vi "Flattening of SGL arrays.vi"() -> ()   [LabVIEW 2017]
uses:
  JSONtext.lvlib
panel:
  in  "enable LabVIEW extensions?":bool=TRUE
  in  "Boolean":bool
  out "time":dbl format="%#_3p"
  out "JSON string":string
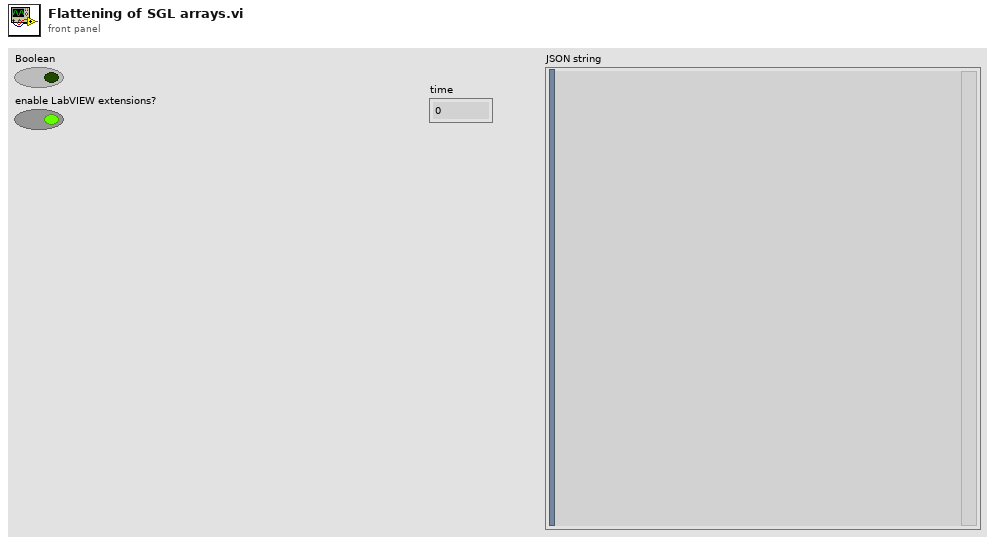
[diagram p1: front panel]
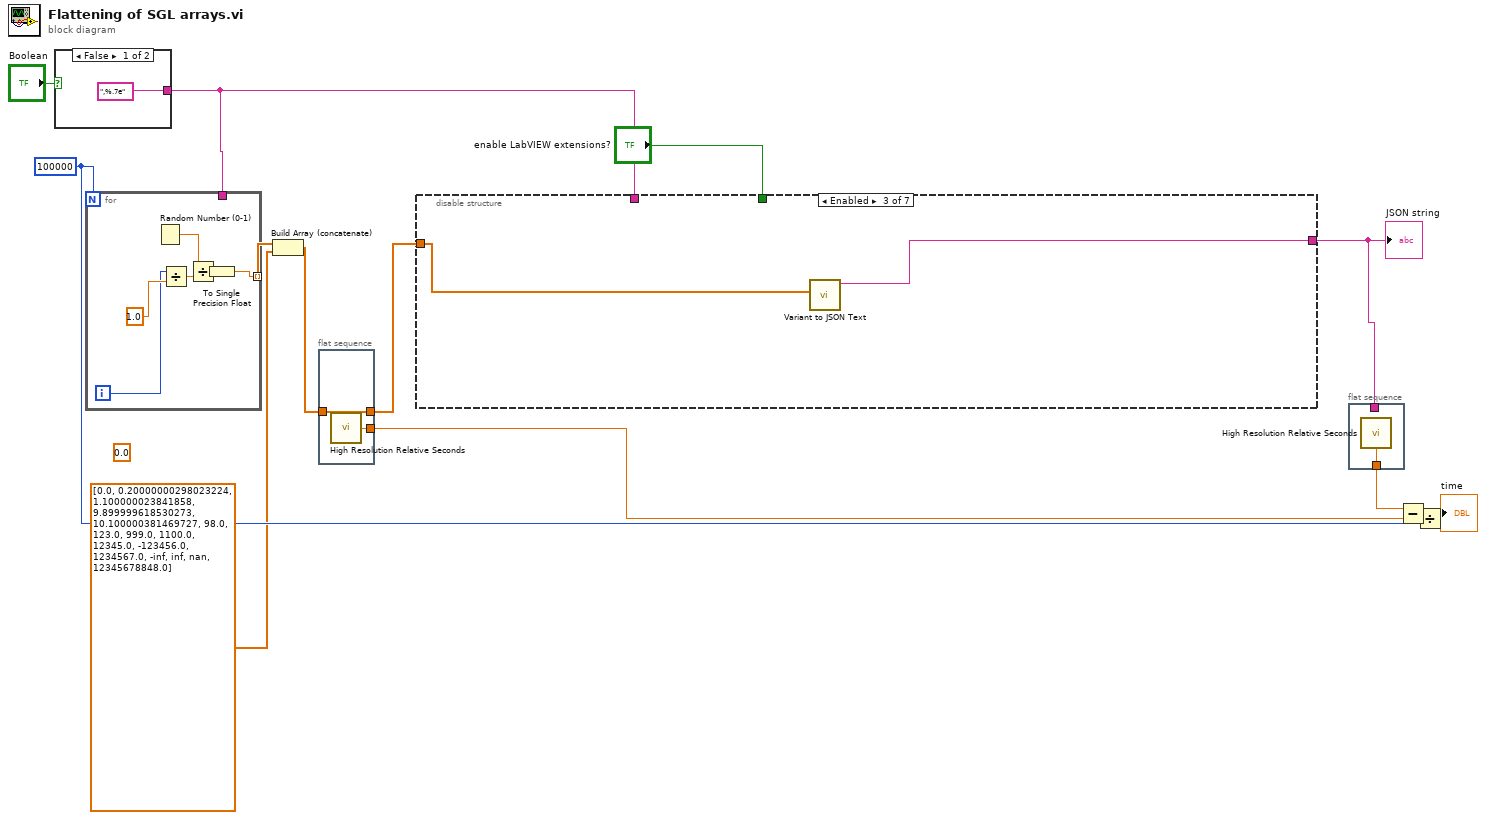
[diagram p0: block diagram]
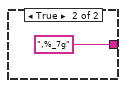
[diagram p2: hidden frame]
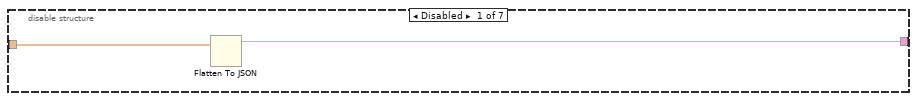
[diagram p3: hidden frame]
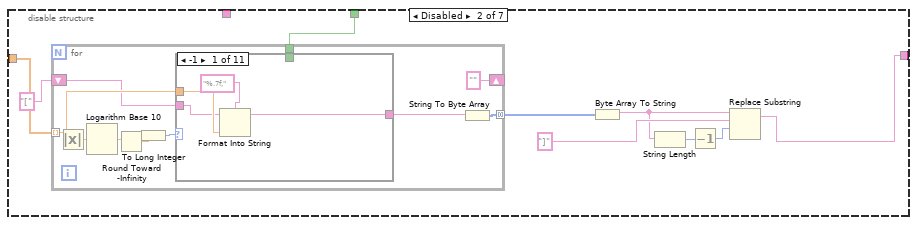
[diagram p4: hidden frame]
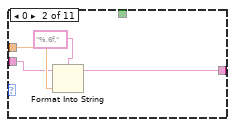
[diagram p5: hidden frame]
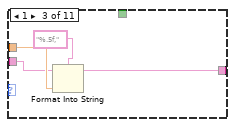
[diagram p6: hidden frame]
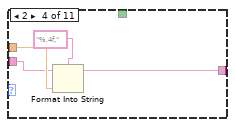
[diagram p7: hidden frame]
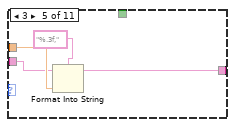
[diagram p8: hidden frame]
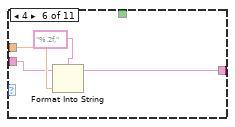
[diagram p9: hidden frame]
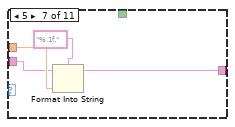
[diagram p10: hidden frame]
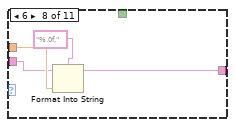
[diagram p11: hidden frame]
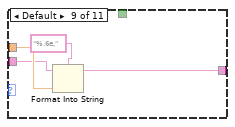
[diagram p12: hidden frame]
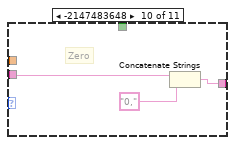
[diagram p13: hidden frame]
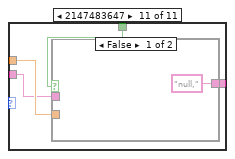
[diagram p14: hidden frame]
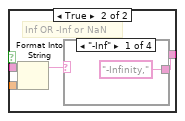
[diagram p15: hidden frame]
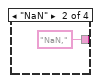
[diagram p16: hidden frame]
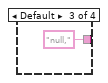
[diagram p17: hidden frame]
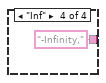
[diagram p18: hidden frame]
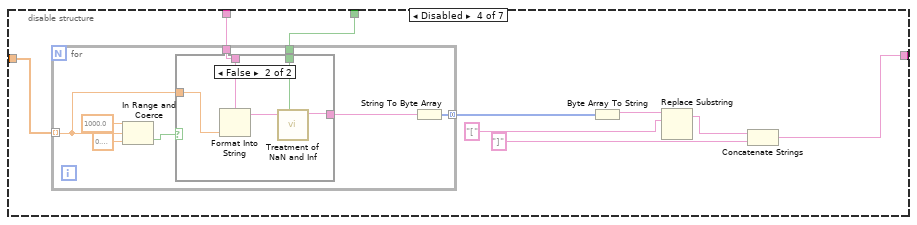
[diagram p19: hidden frame]
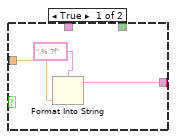
[diagram p20: hidden frame]
diagram:
  (unwired) sgl 0.0
  w6 = 100000
  n1 = case shown="False" "Boolean" {
    tunnel: [",%.7e" ("format string") ",%_7g" ("format string")] -> w3
    frame False {
    }
    frame True {
    }
  }
  n2 = for {
    N: w6 -> [_]
    tunnel: [w16] -> w10 mode=indexing
    tunnel: w3 -> [_]
    i -> [w17]
    n3 = Random Number (0-1)() -> (number: 0 to 1=w19:dbl)
    n4 = Divide(x=w17, y=1.0) -> (x/y=w20:dbl)
    n5 = Divide(x=w19, y=w20) -> (x/y=w18:dbl)
    n6 = To Single Precision Float(number=w18) -> (single precision float=w16:sgl)
  }
  n7 = Build Array (concatenate)(w10, sgl[] [0.0, 0.2, 1.1, 9.9, 10.1, 98.0, 123.0, 999.0, 1100.0, 12345.0, -123456.0, 1234567.0, -inf, inf, nan, 12345679000.0]) -> (w5:sgl[])
  n8 = flat-sequence {
    tunnel: [w23] -> w11
    tunnel: w5 -> [w22]
    tunnel: [w22] -> w9
    frame #0 {
      n9 = call <vilib>:"High Resolution Relative Seconds.vi"() -> ("relative seconds"=w23:dbl)
    }
  }
  n10 = disable-structure shown="Enabled" {
    disable-tunnel: [w25 w30 w97 w101 w126 w141 w164] -> w13
    disable-tunnel: w9 -> [w24 w34 w98 w107 w132 w151 w169]
    disable-tunnel: w3 -> [_ _ _ w100 w125 w139 _]
    disable-tunnel: "enable LabVIEW extensions?" -> [_ w32 _ w99 w124 _ _]
    frame Disabled {
      n11 = Flatten To JSON(anything=w24) -> (JSON string=w25:string)  [unwired: 2 in, 1 out]
    }
    frame Disabled {
      n12 = for {
        tunnel: w34 -> [w42] mode=indexing
        tunnel: [w44] -> w33 mode=concatenating
        tunnel: w32 -> [w43]
        shift-right: [""] -> _
        shift-left: "[" -> [w37]
        n13 = Absolute Value(x=w42) -> (abs(x)=w38:sgl)
        n14 = Logarithm Base 10(1:w38) -> (0:w41:sgl)
        n15 = Round Toward -Infinity(1:w41) -> (0:w40:sgl)
        n16 = To Long Integer(number=w40) -> (32bit integer=w39:i32)
        n17 = case shown="-1" w39 {
          tunnel: [w48 w52 w56 w60 w64 w68 w72 w76 w79 w82 w87] -> w35
          tunnel: w42 -> [w47 w51 w55 w59 w63 w67 w71 w75 w80 _ w86]
          tunnel: w43 -> [_ _ _ _ _ _ _ _ _ _ w85]
          tunnel: w37 -> [w45 w49 w53 w57 w61 w65 w69 w73 w77 w81 w84]
          frame -1 {
            n18 = Format Into String(format string="%.7f,", initial string=w45, w47) -> (resulting string=w48:string)  [unwired: 1 in, 1 out]
          }
          frame 0 {
            n19 = Format Into String(format string="%.6f,", initial string=w49, w51) -> (resulting string=w52:string)  [unwired: 1 in, 1 out]
          }
          frame 1 {
            n20 = Format Into String(format string="%.5f,", initial string=w53, w55) -> (resulting string=w56:string)  [unwired: 1 in, 1 out]
          }
          frame 2 {
            n21 = Format Into String(format string="%.4f,", initial string=w57, w59) -> (resulting string=w60:string)  [unwired: 1 in, 1 out]
          }
          frame 3 {
            n22 = Format Into String(format string="%.3f,", initial string=w61, w63) -> (resulting string=w64:string)  [unwired: 1 in, 1 out]
          }
          frame 4 {
            n23 = Format Into String(format string="%.2f,", initial string=w65, w67) -> (resulting string=w68:string)  [unwired: 1 in, 1 out]
          }
          frame 5 {
            n24 = Format Into String(format string="%.1f,", initial string=w69, w71) -> (resulting string=w72:string)  [unwired: 1 in, 1 out]
          }
          frame 6 {
            n25 = Format Into String(format string="%.0f,", initial string=w73, w75) -> (resulting string=w76:string)  [unwired: 1 in, 1 out]
          }
          frame Default {
            n26 = Format Into String(format string="%.6e,", initial string=w77, w80) -> (resulting string=w79:string)  [unwired: 1 in, 1 out]
          }
          frame -2147483648 {
            # "Zero"
            n27 = Concatenate Strings(w81, "0,") -> (w82:string)
          }
          frame 2147483647 {
            n28 = case shown="False" w85 {
              tunnel: ["null," w92] -> w87
              tunnel: w86 -> [_ w90]
              tunnel: w84 -> [_ w89]
              frame False {
              }
              frame True {
                # "Inf OR -Inf or NaN"
                n29 = Format Into String(initial string=w89, w90) -> (resulting string=w91:string)  [unwired: 2 in, 1 out]
                n30 = case shown="\"-Inf\"" w91 {
                  tunnel: ["-Infinity," "NaN," "null," "-Infinity,"] -> w92
                  frame "-Inf" {
                  }
                  frame "NaN" {
                  }
                  frame Default {
                  }
                  frame "Inf" {
                  }
                }
              }
            }
          }
        }
        n31 = String To Byte Array(string=w35) -> (unsigned byte array=w44:u8[])
      }
      n32 = Byte Array To String(unsigned byte array=w33) -> (string=w28:string)
      n33 = String Length(string=w28) -> (length=w27:i32)
      n34 = Decrement(x=w27) -> (x-1=w26:i32)
      n35 = Replace Substring(3:w26, 4:"]" ("string"), 5:w28) -> (1:w30:string)  [unwired: 1 in, 1 out]
    }
    frame Enabled {
      n36 = call "Variant to JSON Text.vi"("Variant"=w98) -> ("<JSON>"=w97:string)  [unwired: 8 in, 2 out]
    }
    frame Disabled {
      n37 = for {
        tunnel: w107 -> [w109] mode=indexing
        tunnel: [w115] -> w106 mode=concatenating
        tunnel: w100 -> [w114]
        tunnel: w99 -> [w108]
        n38 = In Range and Coerce(upper limit=sgl 1000.0, x=w109, lower limit=sgl 0.1) -> (In Range?=w110:bool)  [unwired: 1 out]
        n39 = case shown="False" w110 {
          tunnel: w114 -> [_ w123]
          tunnel: [w118 w120] -> w113
          tunnel: w109 -> [w117 w122]
          tunnel: w108 -> [_ w119]
          frame True {
            n40 = Format Into String(format string=",%.7f", w117) -> (resulting string=w118:string)  [unwired: 2 in, 1 out]
          }
          frame False {
            n41 = Format Into String(format string=w123, w122) -> (resulting string=w121:string)  [unwired: 2 in, 1 out]
            n42 = call "Treatment of NaN and Inf.vi"("enable LabVIEW extensions?"=w119, "Numeric Text"=w121) -> ("<JSON>"=w120:string)  [unwired: 9 in]
          }
        }
        n43 = String To Byte Array(string=w113) -> (unsigned byte array=w115:u8[])
      }
      n44 = Byte Array To String(unsigned byte array=w106) -> (string=w105:string)
      n45 = Replace Substring(4:"[" ("substring (\"\")"), 5:w105) -> (1:w103:string)  [unwired: 2 in, 1 out]
      n46 = Concatenate Strings(w103, "]" ("string")) -> (w101:string)
    }
    frame Disabled {
      n47 = for {
        tunnel: w132 -> [w138] mode=indexing
        tunnel: [w137] -> w131 mode=concatenating
        tunnel: w125 -> [w136]
        tunnel: w124 -> [w133]
        n48 = Format Into String(format string=w136, w138) -> (resulting string=w135:string)  [unwired: 2 in, 1 out]
        n49 = call "Treatment of NaN and Inf.vi"("enable LabVIEW extensions?"=w133, "Numeric Text"=w135) -> ("<JSON>"=w134:string)  [unwired: 9 in]
        n50 = String To Byte Array(string=w134) -> (unsigned byte array=w137:u8[])
      }
      n51 = Byte Array To String(unsigned byte array=w131) -> (string=w130:string)
      n52 = Replace Substring(4:"[" ("substring (\"\")"), 5:w130) -> (1:w128:string)  [unwired: 2 in, 1 out]
      n53 = Concatenate Strings(w128, "]" ("string")) -> (w126:string)
    }
    frame Disabled {
      n54 = for {
        tunnel: w151 -> [w155] mode=indexing
        tunnel: w139 -> [w154]
        tunnel: [w152] -> w150 mode=indexing
        n55 = Format Into String(format string=w154, w155) -> (resulting string=w153:string)  [unwired: 2 in, 1 out]
        n56 = case shown="\"-Inf\"" w153 {
          selector: w153 -> [_ _ w158]
          tunnel: ["Infinity" "-Infinity" w158] -> w152
          frame "Inf" {
          }
          frame "-Inf" {
          }
          frame Default {
          }
        }
      }
      n57 = Array To Spreadsheet String(delimiter (Tab)=",", array=w150, 3:"" ("format string")) -> (spreadsheet string=w142:string)
      n58 = String Length(string=w142) -> (length=w145:i32)
      n59 = Subtract(x=w145, y=2) -> (x-y=w143:i32)
      n60 = String Subset(string=w142, length (rest)=w143) -> (substring=w146:string)  [unwired: 1 in]
      n61 = Concatenate Strings("[" ("substring (\"\")"), w146, "]" ("substring (\"\")")) -> (w141:string)
    }
    frame Disabled {
      n62 = Array To Spreadsheet String(delimiter (Tab)=",", array=w169, 3:"%#_7g" ("format string")) -> (spreadsheet string=w162:string)
      n63 = String Length(string=w162) -> (length=w161:i32)
      n64 = Subtract(x=w161, y=2) -> (x-y=w159:i32)
      n65 = String Subset(string=w162, length (rest)=w159) -> (substring=w163:string)  [unwired: 1 in]
      n66 = Concatenate Strings("[" ("substring (\"\")"), w163, "]" ("substring (\"\")")) -> (w164:string)
    }
  }
  "JSON string" <- w13
  n67 = flat-sequence {
    tunnel: w13 -> [_]
    tunnel: [w170] -> w12
    frame #0 {
      n68 = call <vilib>:"High Resolution Relative Seconds.vi"() -> ("relative seconds"=w170:dbl)
    }
  }
  n69 = Subtract(x=w12, y=w11) -> (x-y=w8:dbl)
  n70 = Divide(x=w8, y=w6) -> (x/y=→"time":dbl)
